vi "UpdateBooleanRef.vi"(8 "error in (no error)":errorcluster, 11 "AllObjs[]":refnum<vi>[](array[refnum])) -> (0 "error out":errorcluster, 3 "AllObjs[] (dup)":refnum<vi>[](array[refnum]))   [LabVIEW 2017, in "NEVSTOP QD Shortcuts.lvlib"]
uses:
  NEVSTOP QD Shortcuts.lvlib
  <vilib>/Utility/miscctls.llb/LVTextColorsTypeDef.ctl
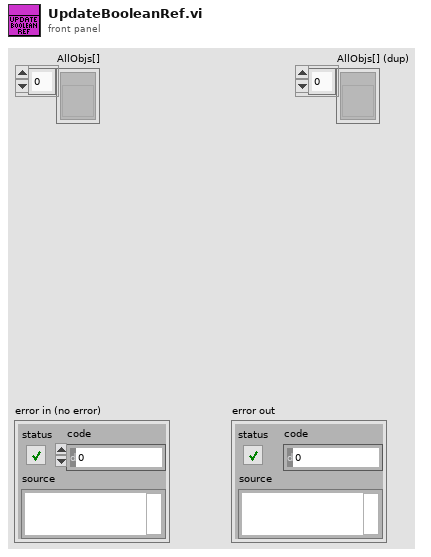
[diagram p1: front panel]
types:
  T1 = typedef "LVTextColorsTypeDef.ctl" = cluster{"Text Color":u32, "Background Color":u32}
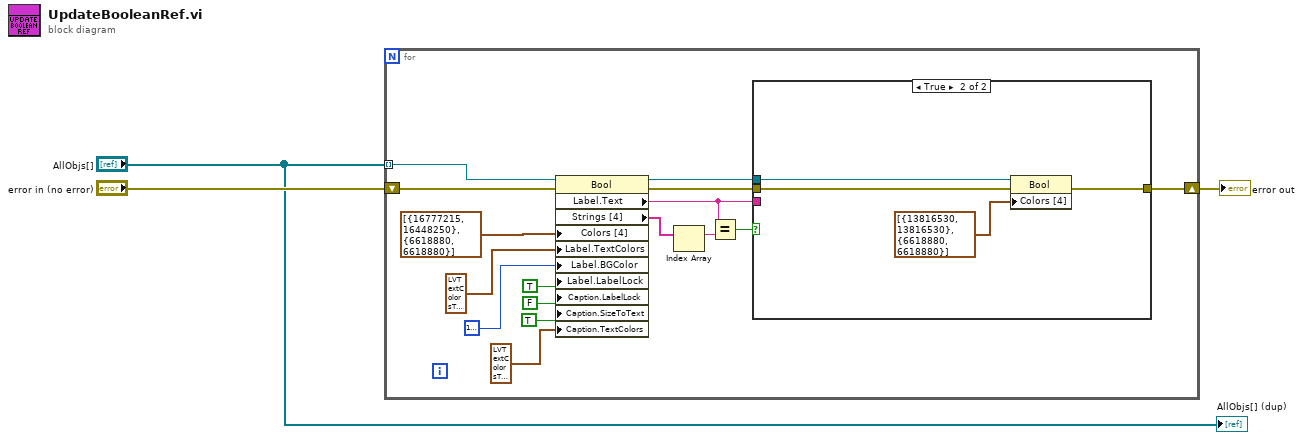
[diagram p0: block diagram]
diagram:
  n1 = for {
    tunnel: "AllObjs[]" -> [w18] mode=indexing
    shift-right: [w15] -> w3
    shift-left: "error in (no error)" -> [w19]
    n2 = property class="Bool"(reference=w18, error in=w19, "Colors [4]"=cluster{u32, u32}[] [{16777215, 16448250}, {6618880, 6618880}], "Label.TextColors"=T1 {"Text Color"=5592405, "Background Color"=5592405} ("Label.Text Colors"), "Label.BGColor"=u32 16777216 ("Text Color"), "Label.LabelLock"=TRUE ("Label.Lock"), "Caption.LabelLock"=FALSE ("Caption.Lock"), "Caption.SizeToText"=TRUE ("Caption.Size to Text?"), "Caption.TextColors"=T1 {"Text Color"=16860, "Background Color"=16777216} ("Label.Text Colors")) -> (reference out=w17:refnum<vi>, error out=w16:errorcluster, "Label.Text"=w14:string, "Strings [4]"=w13:string[])
    n3 = Index Array(array=w13) -> (element=w12:string)  [unwired: 1 in]
    n4 = Equal?(x=w14, y=w12) -> (x = y?=w11:bool)
    n5 = case shown="True" w11 {
      tunnel: w17 -> [_ w24]
      tunnel: w16 -> [w20 w23]
      tunnel: [w20 w22] -> w15
      tunnel: w14 -> [_ _]
      frame False {
      }
      frame True {
        n6 = property class="Bool"(reference=w24, error in=w23, "Colors [4]"=cluster{u32, u32}[] [{13816530, 13816530}, {6618880, 6618880}]) -> (error out=w22:errorcluster)  [unwired: 1 out]
      }
    }
  }
  "error out" <- w3
  "AllObjs[] (dup)" <- "AllObjs[]"
